vi "Make.vi"(8 "error in (no error)":errorcluster, 10 "Msg":string) -> (0 "error out":errorcluster, 3 "Popup Msg out":refnum<class "Popup Msg.lvclass">)   [LabVIEW 2020, in "Test-Client.lvlib" / "Popup Msg.lvclass"]
uses:
  Popup Msg.lvclass
  Popup Msg.lvclass/Popup Msg.ctl
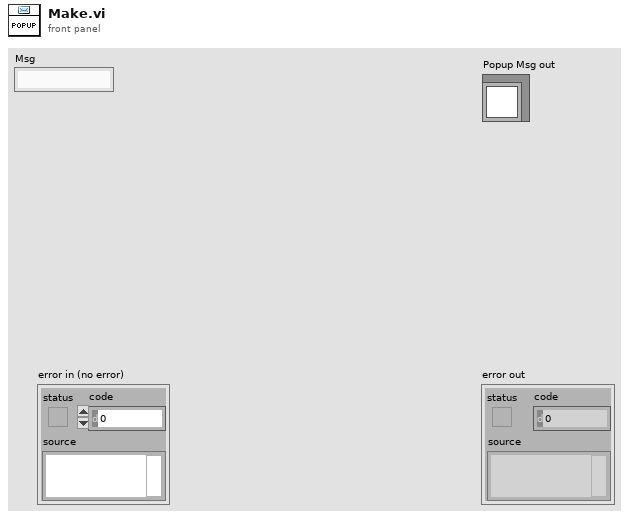
[diagram p1: front panel]
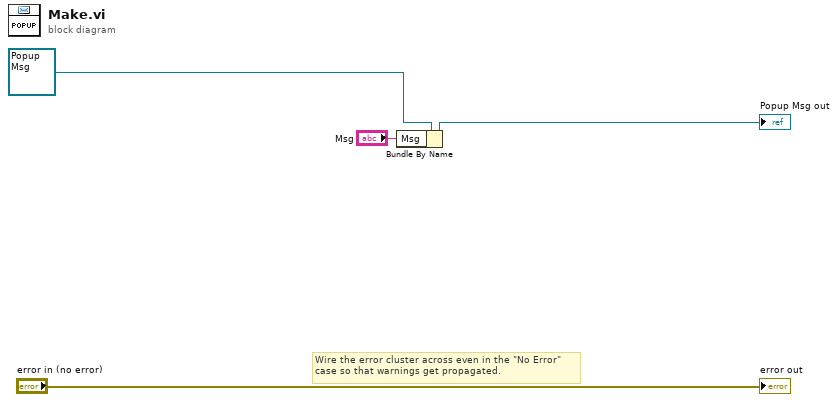
[diagram p0: block diagram]
diagram:
  # "Wire the error cluster across even in the \"No Error\"\ncase so that warnings get propagated."
  n1 = Bundle By Name(cluster=refnum<class "Popup Msg.lvclass"> refnum ("Popup Msg in"), "Msg"="Msg") -> (→"Popup Msg out":refnum<class "Popup Msg.lvclass">)
  "error out" <- "error in (no error)"
